vi "find Age its major or not, Excel sheet , Day 2 (1).vi"() -> ()   [LabVIEW 2025]
uses:
  <vilib>/Utility/file.llb/Read Delimited Spreadsheet (string).vi
  <vilib>/Utility/file.llb/Write Delimited Spreadsheet (string).vi
panel:
  in  "Enum":enum16{"Read", "Write", ""}(ring)
  out "Array":T1(array[cluster])
  out "all rows":string[][](array[string])
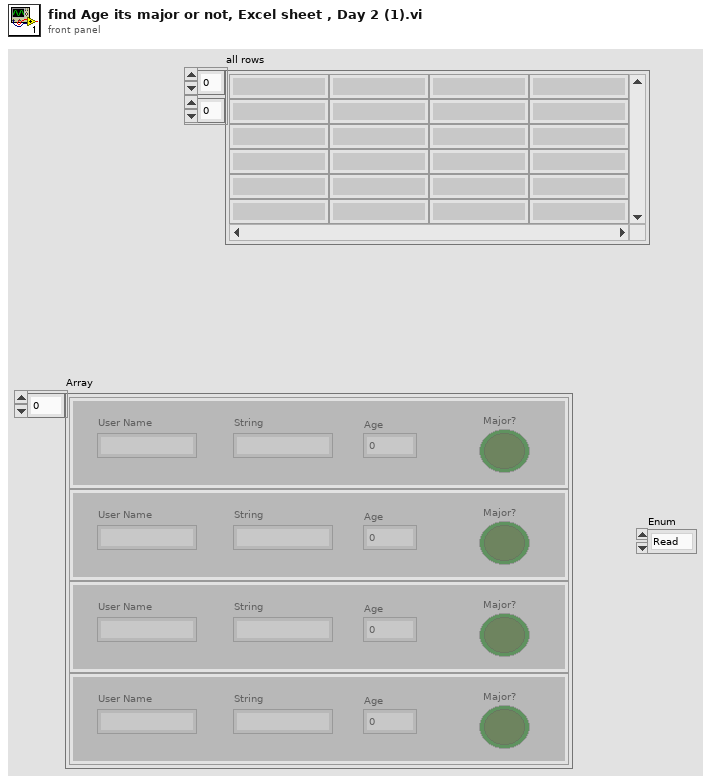
[diagram p1: front panel]
types:
  T1 = cluster{"User Name ":string, "String":string, "Age":dbl, "Major?":bool}[]
  T2 = cluster{"User Name ":string, "String":string, "Age":dbl, "Major?":bool}
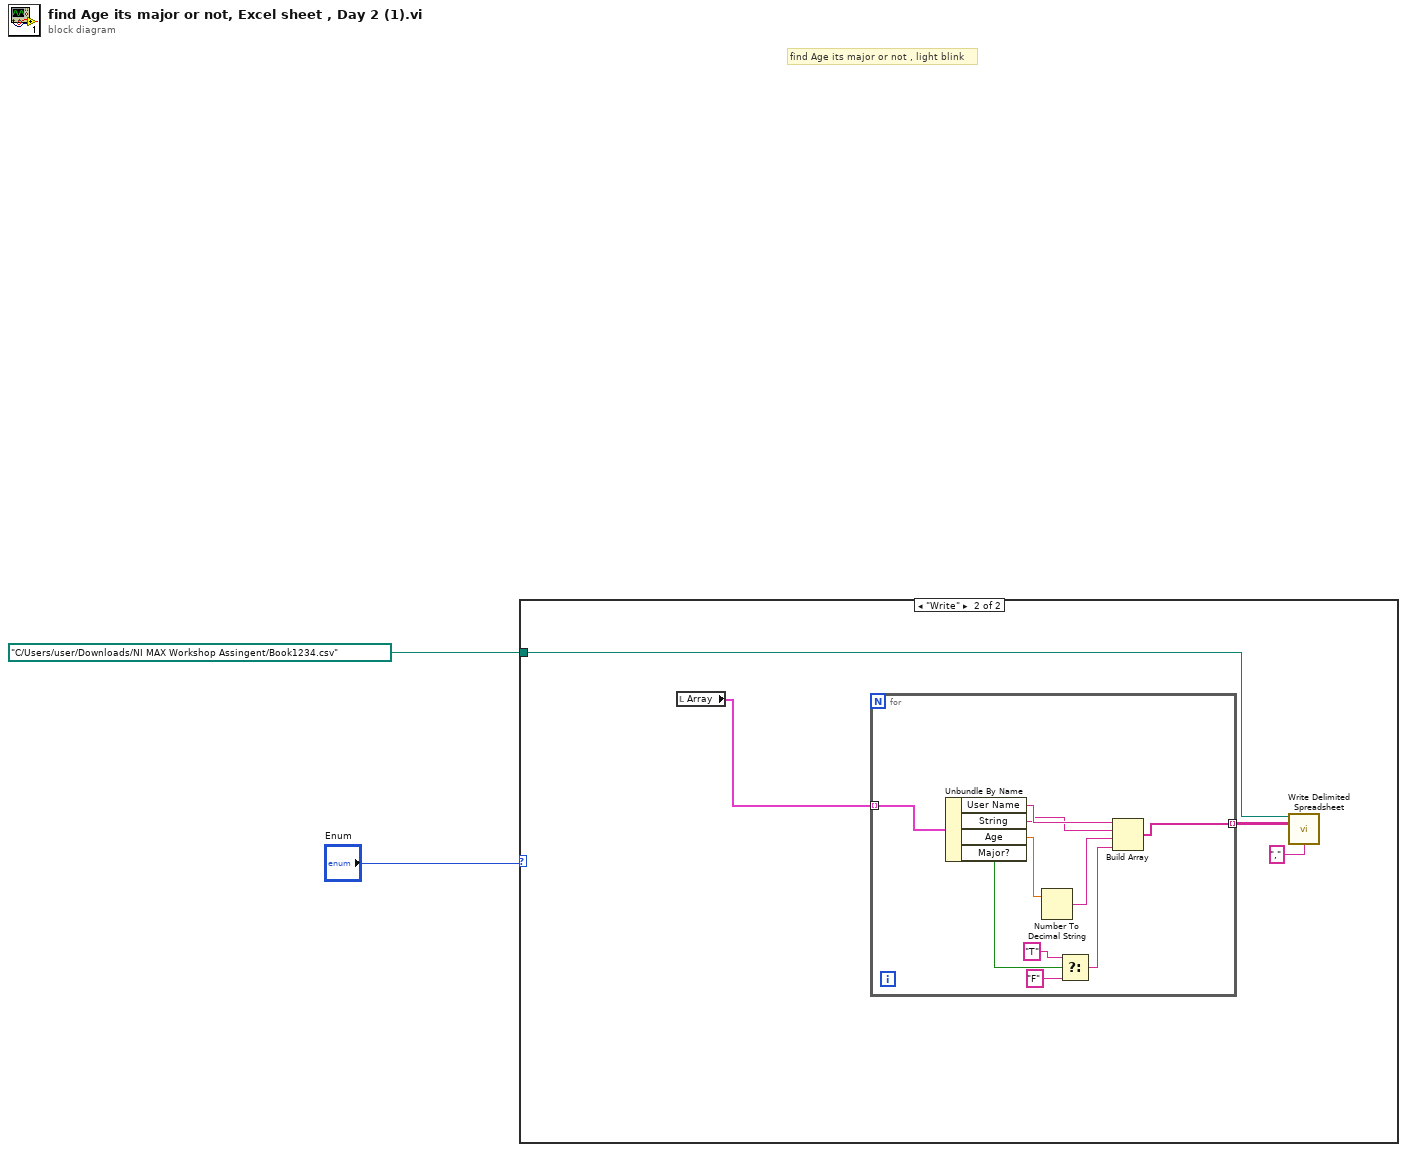
[diagram p0: block diagram]
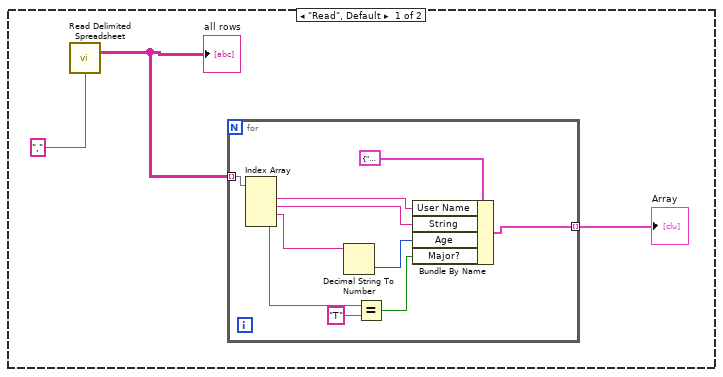
[diagram p2: hidden frame]
diagram:
  # "find Age its major or not , light blink"
  n1 = case shown="\"Write\"" "Enum" {
    tunnel: path "C:/Users/user/Downloads/NI MAX Workshop Assingent/Book1234.csv" ("file path (dialog if empty) 2") -> [_ w16]
    frame "Read", Default {
      n2 = call-poly <vilib>:"Read Delimited Spreadsheet.vi"("delimiter (\\t)"="," ("delimiter (\\t)")) -> ("all rows"=w4:string[][])  [unwired: 9 in, 5 out]
      "all rows" <- w4
      n3 = for {
        tunnel: w4 -> [w15] mode=indexing
        tunnel: [w6] -> w5 mode=indexing
        n4 = Index Array(array=w15) -> (element #1=w8:string, element #2=w9:string, element #3=w12:string, element #4=w11:string)  [unwired: 4 in]
        n5 = Decimal String To Number(string=w12) -> (number=w14:i32)  [unwired: 2 in, 1 out]
        n6 = Equal?(x=w11, y="T") -> (x = y?=w13:bool)
        n7 = Bundle By Name "Bundle By Name"(cluster=T2 {"User Name "="Britto", "String"="12", "Age"=21.0, "Major?"=FALSE} ("Cluster"), "User Name"=w8, "String"=w9, "Age"=w14, "Major?"=w13) -> (w6:T2)
      }
      "Array" <- w5
    }
    frame "Write" {
      n8 = local read "Array"() -> (w19:T1)
      n9 = for {
        tunnel: w19 -> [w29] mode=indexing
        tunnel: [w22] -> w18 mode=indexing
        n10 = Unbundle By Name(w29) -> ("User Name"=w28:string, "String"=w27:string, "Age"=w26:dbl, "Major?"=w24:bool)
        n11 = Number To Decimal String(number=w26) -> (decimal integer string=w25:string)  [unwired: 1 in]
        n12 = Select(t="T", s=w24, f="F") -> (s? t:f=w23:string)
        n13 = Build Array(w28, w27, w25, w23) -> (w22:string[])
      }
      n14 = call-poly <vilib>:"Write Delimited Spreadsheet.vi"("file path (dialog if empty)"=w16, "2D data"=w18, "delimiter (\\t)"="," ("delimiter (\\t)")) -> ()  [unwired: 11 in, 2 out]
    }
  }
